vi "Write FPGATarget.lvclass.vi"(8 "error in (no error)":errorcluster, 10 "FPGATarget.lvclass":refnum<class "FPGATarget.lvclass">, 11 "FPGASession in":refnum<class "FPGASession.lvclass">) -> (0 "error out":errorcluster, 3 "FPGASession out":refnum<class "FPGASession.lvclass">)   [LabVIEW 2013, in "FPGASession.lvclass"]
uses:
  FPGASession.lvclass
  FPGATargetClass/FPGATarget.lvclass
  FPGASession.lvclass/FPGASession.ctl
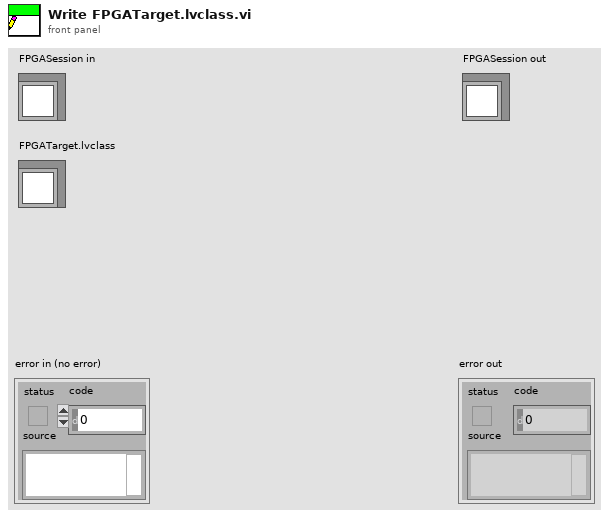
[diagram p1: front panel]
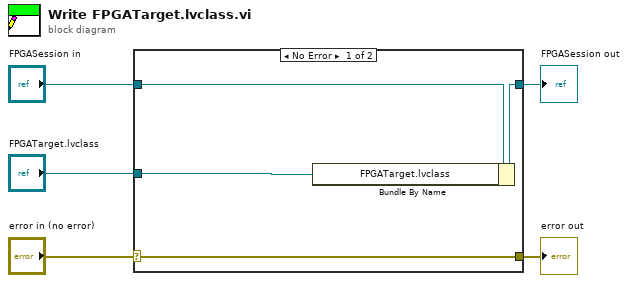
[diagram p0: block diagram]
diagram:
  n1 = case shown="No Error" "error in (no error)" {
    selector: "error in (no error)" -> [w9 w10]
    tunnel: [w9 w10] -> w4
    tunnel: [w7 w11] -> w2
    tunnel: "FPGASession in" -> [w8 w11]
    tunnel: "FPGATarget.lvclass" -> [w6 _]
    frame No Error {
      n2 = Bundle By Name(cluster=w8, "FPGATarget.lvclass"=w6) -> (w7:refnum<class "FPGASession.lvclass">)
    }
    frame Error {
    }
  }
  "error out" <- w4
  "FPGASession out" <- w2
